vi "Load DAC Configuration.vi"(8 "error in":errorcluster, 10 "Config File refnum in":T1, 11 "DAC Inclino in":refnum<class "DAC Inclinometer.lvclass">) -> (0 "error out":errorcluster, 2 "Config File refnum out":T1, 3 "DAC Inclino out":refnum<class "DAC Inclinometer.lvclass">)   [LabVIEW 2019, in "DAC.lvlib" / "DAC Inclinometer.lvclass"]
uses:
  DAC Inclinometer.lvclass
  <vilib>/Utility/config.llb/Config Data RefNum.ctl
  DAC.lvclass
  <vilib>/Utility/config.llb/NI_LVConfig.lvlib
  <vilib>/Utility/config.llb/Read Key (Double).vi
  C:/Users/wg/Documents/LV_Projects/test-stand/App/DAC/DAC.lvclass
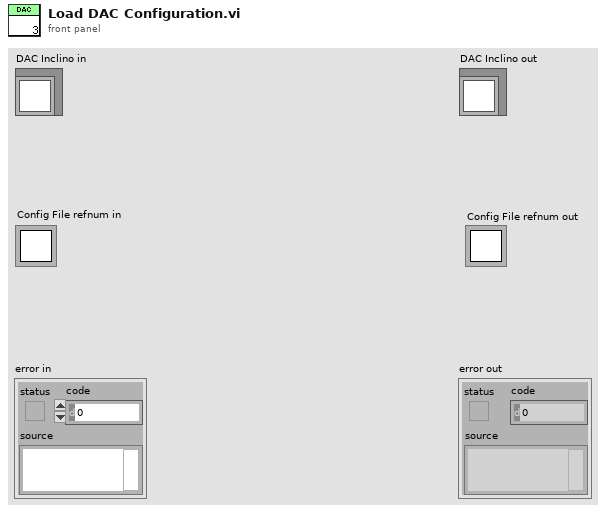
[diagram p1: front panel]
types:
  T1 = typedef "NI_LVConfig.lvlib/Config Data RefNum.ctl" = refnum<k1>
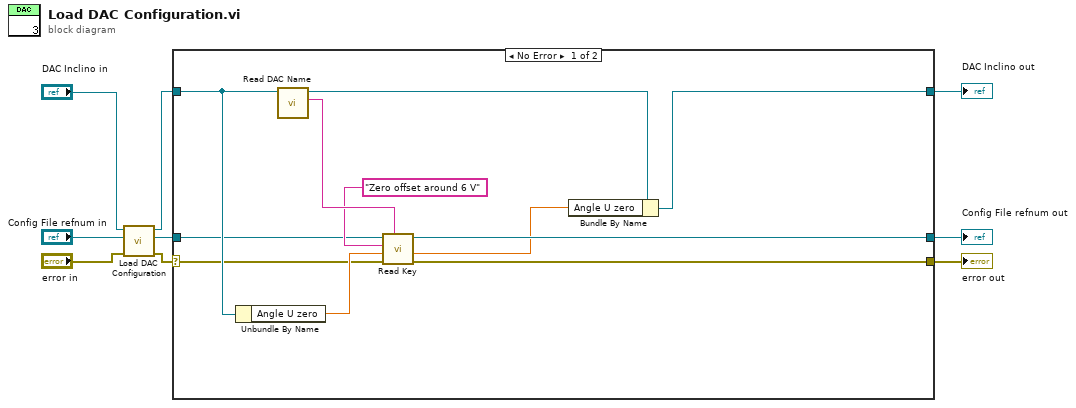
[diagram p0: block diagram]
diagram:
  n1 = call-parent "Load DAC Configuration.vi"("error in"="error in", "Config File refnum in"="Config File refnum in", "DAC in"="DAC Inclino in") -> ("error out"=w4:errorcluster, "Config File refnum out"=w5:T1, "DAC out"=w6:refnum<class "DAC Inclinometer.lvclass">)  [unwired: 6 in]
  n2 = case shown="No Error" w4 {
    selector: w4 -> [w15 w23]
    tunnel: [w11 w23] -> w1
    tunnel: [w13 w22] -> w3
    tunnel: w6 -> [w17 w22]
    tunnel: w5 -> [w16 w21]
    tunnel: [w12 w21] -> w2
    frame No Error {
      n3 = Unbundle By Name(w17) -> ("Angle U zero"=w18:dbl)
      n4 = call "Read DAC Name.vi"("DAC in"=w17) -> ("DAC Name"=w20:string, "DAC out"=w14:refnum<class "DAC Inclinometer.lvclass">)  [unwired: 8 in, 1 out]
      n5 = call-poly <vilib>:"Read Key.vi"("section"=w20, "error in (no error)"=w15, "default value"=w18, "key"="Zero offset around 6 V", "refnum"=w16) -> ("error out"=w11:errorcluster, "value"=w10:dbl, "refnum out"=w12:T1)  [unwired: 3 in, 1 out]
      n6 = Bundle By Name(cluster=w14, "Angle U zero"=w10) -> (w13:refnum<class "DAC Inclinometer.lvclass">)
    }
    frame Error {
    }
  }
  "error out" <- w1
  "DAC Inclino out" <- w3
  "Config File refnum out" <- w2
